vi "Cryostat.vi"(8 "error in (no error)":errorcluster, 11 "Cryostat in":refnum<class "Cryostat.lvclass">) -> (0 "error out":errorcluster, 3 "Cryostat out":refnum<class "Cryostat.lvclass">)   [LabVIEW 2017, in "Cryostat.lvclass"]
uses:
  Cryostat.lvclass
  C:/LabVIEW-programs/Instruments/Utility Classes/Readable/Readable.lvclass
  Global/GPIB Numbers.vi
  Utility Classes/Readable/Readable.lvclass
panel:
  out "Status":string
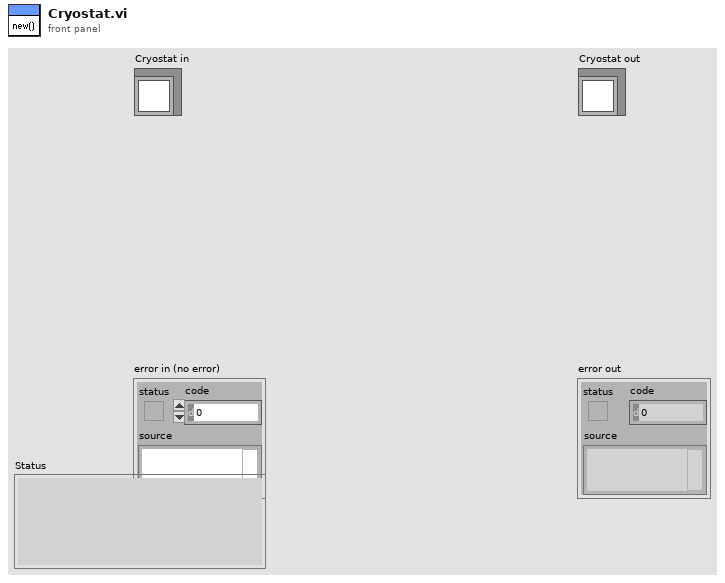
[diagram p1: front panel]
types:
  T1 = typedef "GPIB Type Def.ctl" = cluster{"Name":string, "bus":dbl, "GPIB":dbl, "GPIB as string":string, "byte":i32, "VISA Resource Name":refnum<visa-resource-name>}
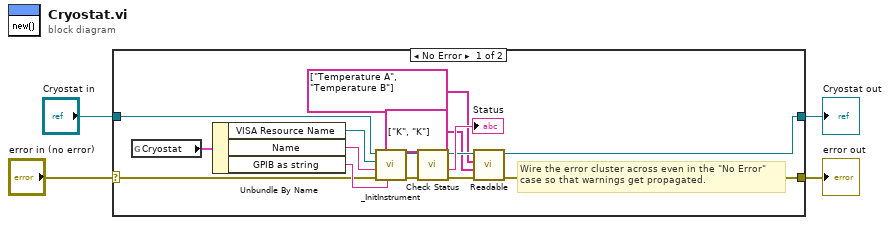
[diagram p0: block diagram]
diagram:
  n1 = case shown="No Error" "error in (no error)" {
    selector: "error in (no error)" -> [w6 w21]
    tunnel: [w5 w21] -> w3
    tunnel: [w7 w20] -> w1
    tunnel: "Cryostat in" -> [w8 w20]
    frame No Error {
      # "Wire the error cluster across even in the \"No Error\"\ncase so that warnings get propagated."
      n2 = global read "GPIB Numbers.vi" "Cryostat"() -> (w19:T1)
      n3 = Unbundle By Name(w19) -> ("VISA Resource Name"=w17:refnum<visa-resource-name>, "Name"=w16:string, "GPIB as string"=w15:string)
      n4 = call-dynamic "_InitInstrument.vi"("GPIB as string"=w15, "error in (no error)"=w6, "Name"=w16, "VISA Resource Name"=w17, "Instrument in"=w8) -> ("error out"=w14:errorcluster, "Instrument out"=w18:refnum<class "Cryostat.lvclass">)  [unwired: 1 in, 4 out]
      n5 = call-dynamic "Check Status.vi"("error in (no error)"=w14, "Cryostat in"=w18) -> ("error out"=w12:errorcluster, "Status"=→"Status":string, "Cryostat out"=w11:refnum<class "Cryostat.lvclass">)  [unwired: 7 out]
      n6 = call "Readable.vi"("error in (no error)"=w12, "Channel Units"=string[] ["K", "K"], "Channel Names"=string[] ["Temperature A", "Temperature B"], "Readable in"=w11) -> ("error out"=w5:errorcluster, "Readable out"=w7:refnum<class "Cryostat.lvclass">)  [unwired: 6 in]
    }
    frame Error {
    }
  }
  "error out" <- w3
  "Cryostat out" <- w1
